vi "SetEventData Example.vi"() -> ()   [LabVIEW 2010]
uses:
  <vilib>/builds/MDSplus/MDSplus/MDSplus.lvlib
panel:
  in  "Event Data":i32
  in  "Event Name":string="CACCOLA"
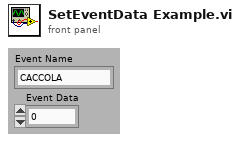
[diagram p1: front panel]
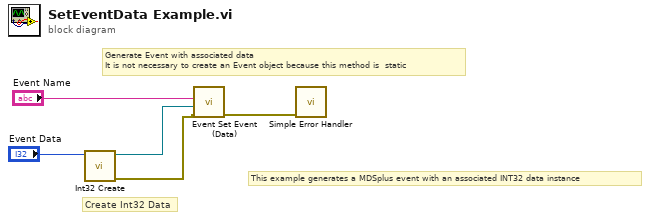
[diagram p0: block diagram]
diagram:
  # "This example generates a MDSplus event with an associated INT32 data instance"
  # "Generate Event with associated data\nIt is not necessary to create an Event object because this method is  static"
  # "Create Int32 Data"
  n1 = call <vilib>:"Int32 Create.vi"("I32 in"="Event Data") -> ("error out"=w2:errorcluster, "Int32 DVR out"=w3:refnum<data-value>)  [unwired: 9 in]
  n2 = call <vilib>:"Event Set Event (Data).vi"("error in (no error)"=w2, "Data"=w3, "Event name"="Event Name") -> ("error out"=w1:errorcluster)  [unwired: 7 in, 1 out]
  n3 = call <vilib>:"Simple Error Handler.vi"("error in (no error)"=w1) -> ()  [unwired: 4 in, 5 out]
